vi "LVUT_MainSequence(Multisocket Example_Station1).vi"(8 "error in (no error)":errorcluster) -> (0 "error out":errorcluster)   [LabVIEW 2019, in "Multisocket Example(Station1).lvlib"]
uses:
  Multisocket Example(Station1).lvlib
  Unit Test Engine Tools.lvlib
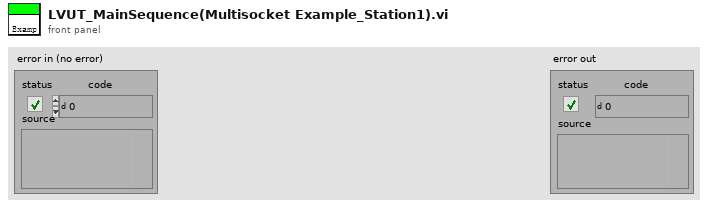
[diagram p1: front panel]
types:
  T1 = enum16{"Station 1", "Station 2", "Station 3", "Station 4"}
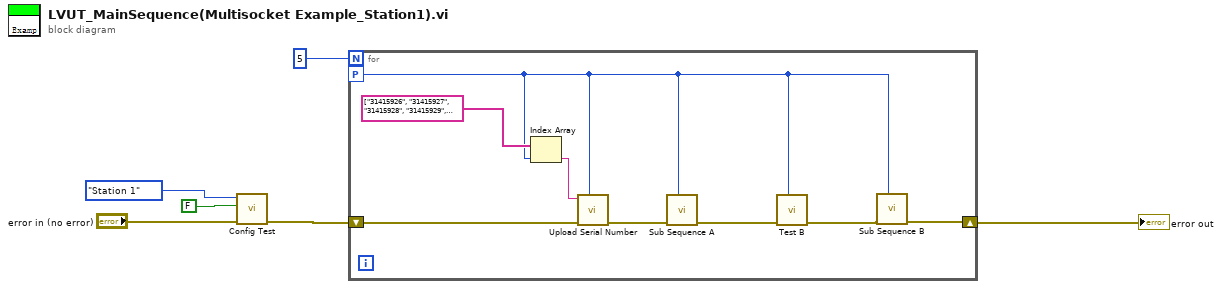
[diagram p0: block diagram]
diagram:
  n1 = call "Config Test.vi"("Error In"="error in (no error)", "Debug"=FALSE, "Station"=T1."Station 1") -> ("Error Out"=w1:errorcluster)  [unwired: 8 in]
  n2 = for {
    N: 5 -> [_]
    shift-right: [w12] -> w3
    shift-left: w1 -> [w10]
    workers-P: _ -> [w8]
    n3 = Index Array(array=string[] ["31415926", "31415927", "31415928", "31415929", "31415930"], index=w8) -> (element=w7:string)
    n4 = call "Upload Serial Number.vi"("Socket"=w8, "error in (no error)"=w10, "SerialNumber"=w7) -> ("error out"=w11:errorcluster)  [unwired: 8 in]
    n5 = call "Sub Sequence A.vi"("Socket"=w8, "error in (no error)"=w11) -> ("error out"=w13:errorcluster)  [unwired: 9 in]
    n6 = call "Test B.vi"("Socket"=w8, "error in (no error)"=w13) -> ("error out"=w14:errorcluster)  [unwired: 9 in]
    n7 = call "Sub Sequence B.vi"("Socket"=w8, "error in (no error)"=w14) -> ("error out"=w12:errorcluster)  [unwired: 9 in]
  }
  "error out" <- w3
